vi "BuildPresentPicture.vi"(0 "Desired Dimensions":cluster{"Width":i32, "Height":i32}={"Width"=320, "Height"=240}, 1 "Pict Refnum":refnum<vi>) -> (2 "Valid slides?":bool, 3 "SlideInfo":T1[](array[typedef]))   [LabVIEW 2012]
uses:
  SlideTypeDef.ctl
  <vilib>/Utility/miscctls.llb/LVPointTypeDef.ctl
  SlideParams.ctl
  <vilib>/Utility/file.llb/Read From Spreadsheet File (string).vi
  LVPresent_Globals.vi
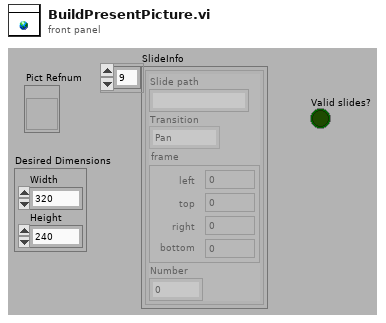
[diagram p1: front panel]
types:
  T1 = typedef "SlideTypeDef.ctl" = cluster{"Slide path":string, "Transition":enum16{"Pan", "Zoom-pan-zoom", "Zoom-wait-Zoom"}, "frame":cluster{"left":i16, "top":i16, "right":i16, "bottom":i16}, "Number":i32}
  T2 = typedef "LVPointTypeDef.ctl" = cluster{"Horizontal":i16, "Vertical":i16}
  T3 = typedef "SlideParams.ctl" = enum32{"No Selection", "Bounce", "Order", "Hide", "Remove"}
  T4 = typedef "ParamterCluster.ctl" = cluster{"bounce?":bool, "black?":bool, "slide number":i32, "hide?":bool, "selection":bool}
  T5 = cluster{"left":i16, "top":i16, "right":i16, "bottom":i16}
  T6 = cluster{"file name":string, "Transition":enum16{"Pan", "Zoom-pan-zoom"}, "frame":cluster{"left":i16, "top":i16, "right":i16, "bottom":i16}, "slide number":i32}
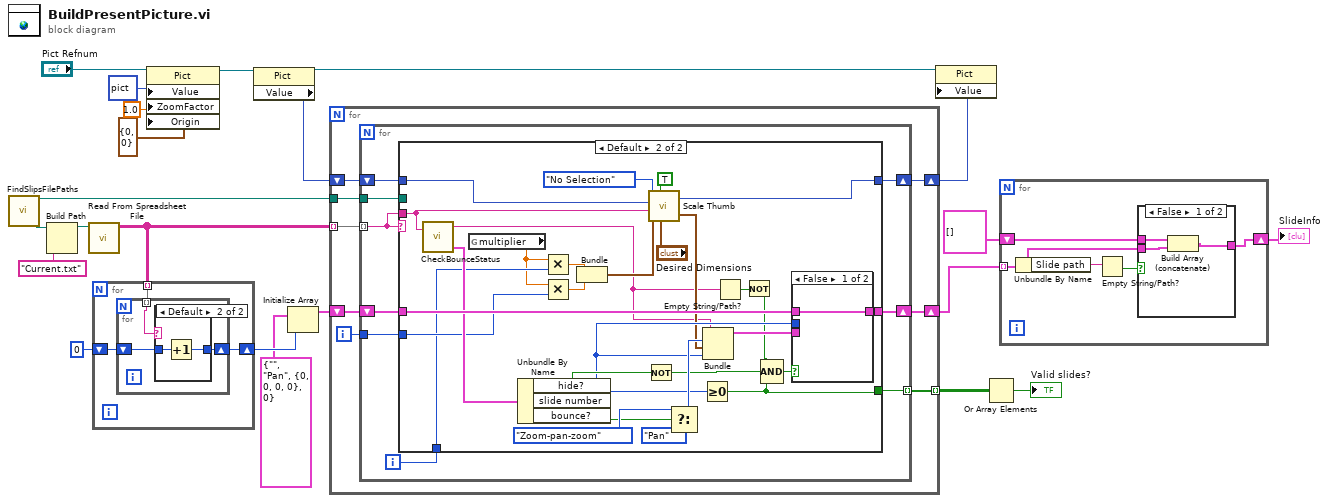
[diagram p0: block diagram]
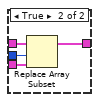
[diagram p5: hidden frame]
diagram:
  n1 = call "FindSlipsFilePaths.vi"() -> ("Playlists"=w21:path, "Slides"=w22:path)  [unwired: 2 in, 3 out]
  n2 = Build Path(base path=w21, name or relative path="Current.txt") -> (appended path=w19:path)
  n3 = call-poly <vilib>:"Read From Spreadsheet File.vi"("file path (dialog if empty)"=w19) -> ("all rows"=w18:string[][])  [unwired: 6 in, 4 out]
  n4 = for {
    tunnel: w18 -> [w25] mode=indexing
    shift-right: [w24] -> w16
    shift-left: 0 -> [w23]
    n5 = for {
      tunnel: w25 -> [w28] mode=indexing
      shift-right: [w27] -> w24
      shift-left: w23 -> [w26]
      n6 = case shown="Default" w28 {
        tunnel: [w29 w31] -> w27
        tunnel: w26 -> [w29 w30]
        frame "" {
        }
        frame Default {
          n7 = Increment(x=w30) -> (x+1=w31:i32)
        }
      }
    }
  }
  n8 = property class="Pict"(reference="Pict Refnum", "Value"=picture data[5B], "ZoomFactor"=sgl 1.0 ("Zoom Factor"), "Origin"=T2 {"Horizontal"=0, "Vertical"=0}) -> (reference out=w1:refnum<vi>)  [unwired: 1 in, 1 out]
  n9 = property class="Pict"(reference=w1) -> (reference out=w6:refnum<vi>, "Value"=w8:picture)  [unwired: 1 in, 1 out]
  n10 = Initialize Array(T1 {"Slide path"="", "Transition"=enum."Pan", "frame"={"left"=0, "top"=0, "right"=0, "bottom"=0}, "Number"=0}, w16) -> (w15:T1[])
  n11 = for {
    tunnel: w18 -> [w39] mode=indexing
    tunnel: w22 -> [w38]
    shift-right: [w36] -> w11
    shift-left: w15 -> [w35]
    tunnel: [w34] -> w13 mode=indexing
    shift-right: [w32] -> w7
    shift-left: w8 -> [w33]
    i -> [w37]
    n12 = for {
      tunnel: w38 -> [w48]
      tunnel: w39 -> [w45] mode=indexing
      tunnel: w37 -> [w47]
      shift-right: [w44] -> w36
      shift-left: w35 -> [w43]
      tunnel: [w42] -> w34 mode=indexing
      shift-right: [w40] -> w32
      shift-left: w33 -> [w41]
      i -> [w46]
      n13 = case shown="Default" w45 {
        tunnel: w48 -> [_ _]
        tunnel: w45 -> [_ w55]
        tunnel: w47 -> [_ w57]
        tunnel: w46 -> [_ w56]
        tunnel: [w50 w74] -> w44
        tunnel: w43 -> [w50 w75]
        tunnel: [_ w62] -> w42
        tunnel: w41 -> [w49 w52]
        tunnel: [w49 w51] -> w40
        frame "" {
        }
        frame Default {
          n14 = call "CheckBounceStatus.vi"("File Name"=w55) -> ("Parameters"=w70:T4, "file name"=w60:string)  [unwired: 1 in, 1 out]
          n15 = global read "LVPresent_Globals.vi" "multiplier"() -> (w53:sgl)
          n16 = Unbundle By Name(w70) -> ("hide?"=w72:bool, "slide number"=w71:i32, "bounce?"=w76:bool)
          n17 = Multiply(x=w53, y=w56) -> (x*y=w68:sgl)
          n18 = Multiply(x=w53, y=w57) -> (x*y=w67:sgl)
          n19 = Bundle(w68, w67) -> (w66:cluster{sgl, sgl})  [unwired: 1 in]
          n20 = Not(x=w72) -> (.not. x?=w63:bool)
          n21 = call "Scale Thumb.vi"("Desired Dimensions"="Desired Dimensions", "Full Size"=TRUE ("Show Labels"), "Offset"=w66, "file"=w55, "picture in"=w52, "Mod"=SlideParams."No Selection") -> ("frame"=w64:T5, "new picture"=w51:picture)
          n22 = Select(t=enum16{"Pan", "Zoom-pan-zoom"}."Zoom-pan-zoom" ("Transition"), s=w76, f=enum16{"Pan", "Zoom-pan-zoom"}."Pan" ("Transition")) -> (s? t:f=w77:enum16{"Pan", "Zoom-pan-zoom"})
          n23 = Greater Or Equal To 0?(x=w71) -> (x >= 0?=w62:bool)
          n24 = Bundle("file name"=w60, "Transition"=w77, "frame"=w64, "slide number"=w71) -> (w73:T6)  [unwired: 1 in]
          n25 = Empty String/Path?(string/path=w60) -> (empty?=w59:bool)
          n26 = Not(x=w59) -> (.not. x?=w58:bool)
          n27 = Compound Arithmetic op=AND(w58, w63, w62) -> (w61:bool)
          n28 = case shown="False" w61 {
            tunnel: w75 -> [w80 w84]
            tunnel: [w80 w83] -> w74
            tunnel: w73 -> [_ w81]
            tunnel: w71 -> [_ w82]
            frame False {
            }
            frame True {
              n29 = Replace Array Subset(array=w84, new element=w81, index=w82) -> (w83:T1[])
            }
          }
        }
      }
    }
  }
  n30 = property class="Pict"(reference=w6, "Value"=w7) -> ()  [unwired: 1 in, 2 out]
  n31 = Or Array Elements(Boolean array=w13) -> (logical OR=→"Valid slides?":bool)
  n32 = for {
    shift-right: [w85] -> w9
    shift-left: T1[] [] -> [w86]
    tunnel: w11 -> [w87] mode=indexing
    n33 = Unbundle By Name(w87) -> ("Slide path"=w89:string)
    n34 = Empty String/Path?(string/path=w89) -> (empty?=w88:bool)
    n35 = case shown="False" w88 {
      tunnel: w87 -> [w92 _]
      tunnel: w86 -> [w91 w93]
      tunnel: [w90 w93] -> w85
      frame False {
        n36 = Build Array (concatenate)(w91, w92) -> (w90:T1[])
      }
      frame True {
      }
    }
  }
  "SlideInfo" <- w9
